vi "testWriteToExistingFileFailsWithError.vi"(8 "error in (no error)":errorcluster, 11 "TestCase in":refnum<class "EasyXMLTest.lvclass">) -> (0 "error out":errorcluster, 3 "TestCase out":refnum<class "EasyXMLTest.lvclass">)   [LabVIEW 2013, in "EasyXMLTest.lvclass"]
doc: "This tests whether writing to an existing file generates an error."
uses:
  EasyXMLTest.lvclass
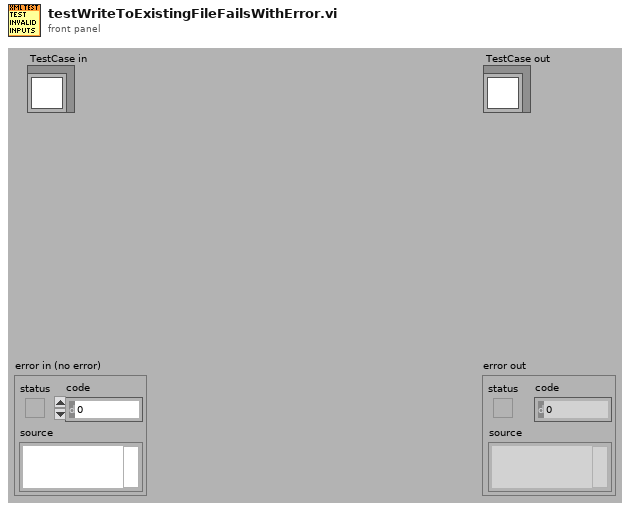
[diagram p1: front panel]
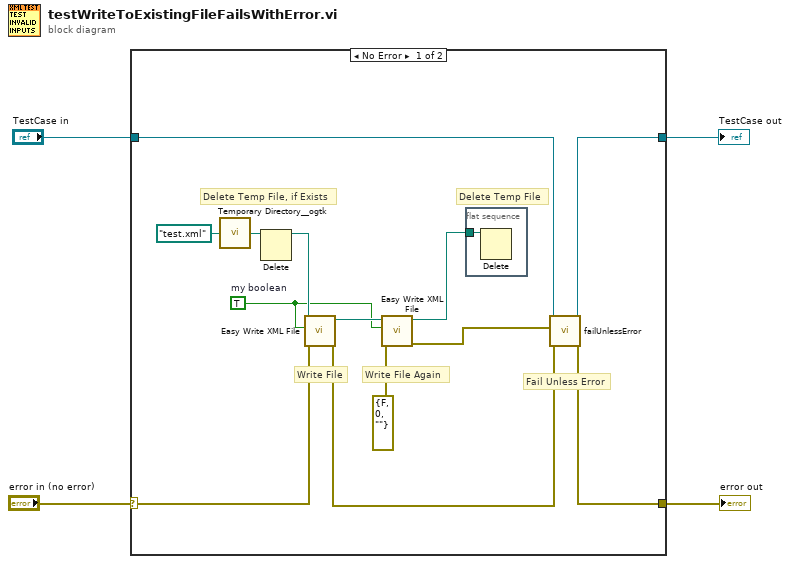
[diagram p0: block diagram]
diagram:
  n1 = case shown="No Error" "error in (no error)" {
    selector: "error in (no error)" -> [w17 w20]
    tunnel: [w9 w20] -> w3
    tunnel: [w7 w19] -> w1
    tunnel: "TestCase in" -> [w8 w19]
    frame No Error {
      w5 = TRUE  # my boolean
      # "Fail Unless Error"
      # "Write File Again"
      # "Write File"
      # "Delete Temp File"
      # "Delete Temp File, if Exists"
      n2 = call <userlib>:"Temporary Directory__ogtk.vi"("Relative path (.)"=path "test.xml") -> ("Temporary Directory (+ Relative)"=w15:path)
      n3 = Delete(path (use dialog)=w15) -> (deleted path=w14:path)  [unwired: 4 in, 2 out]
      n4 = call "Easy Write XML File.vi"("error in (no error)"=w17, "LabVIEW Data"=w5, "XML File Path"=w14) -> ("error out"=w10:errorcluster, "XML File Path (duplicate)"=w13:path)  [unwired: 7 in]
      n5 = call "Easy Write XML File.vi"("error in (no error)"=errorcluster {"status"=FALSE, "code"=0, "source"=""}, "LabVIEW Data"=w5, "XML File Path"=w13) -> ("error out"=w11:errorcluster, "XML File Path (duplicate)"=w12:path)  [unwired: 7 in]
      n6 = flat-sequence {
        tunnel: w12 -> [w18]
        frame #0 {
          n7 = Delete(path (use dialog)=w18) -> ()  [unwired: 4 in, 3 out]
        }
      }
      n8 = call-dynamic "failUnlessError.vi"("error in (no error)"=w10, "error"=w11, "TestCase in"=w8) -> ("error out"=w9:errorcluster, "TestCase out"=w7:refnum<class "EasyXMLTest.lvclass">)  [unwired: 7 in]
    }
    frame Error {
    }
  }
  "error out" <- w3
  "TestCase out" <- w1
